vi "New from MsgPack bytes.vi"(8 "error in (no error)":errorcluster, 11 "Bytes in":u8[](array[numeric]) format="%x") -> (0 "error out":errorcluster, 2 "MsgPackExt":refnum<class "MsgPackExt.lvclass">, 3 "remaining bytes":u8[](array[numeric]))   [LabVIEW 2020, in "MessagePack.lvlib" / "MsgPackExt.lvclass"]
uses:
  MsgPackExt.lvclass
  MsgPackExt.lvclass/MsgPackExt.ctl
  <vilib>/Utility/error.llb/Error Cluster From Error Code.vi
  <vilib>/ErrorRing/Error Ring.xnode
  MessagePack.lvlib
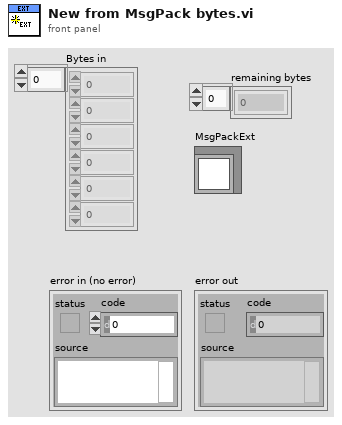
[diagram p1: front panel]
types:
  T1 = typedef "MessagePack.lvlib/MsgPack Object Types.ctl" = enum16{"UNSUPPORTED", "POSINT", "NEGINT", "FIXMAP", "FIXARRAY", "FIXSTR", "NIL", "FALSE", "TRUE", "BIN8", "BIN16", "BIN32", "EXT8", "EXT16", "EXT32", "FLOAT32", "FLOAT64", "UINT8", "UINT16", "UINT32", "UINT64", "INT8", "INT16", "INT32", "INT64", "FIXEXT1", "FIXEXT2", "FIXEXT4", "FIXEXT8", "FIXEXT16", "STR8", "STR16", "STR32", "ARRAY16", "ARRAY32", "MAP16", "MAP32"}
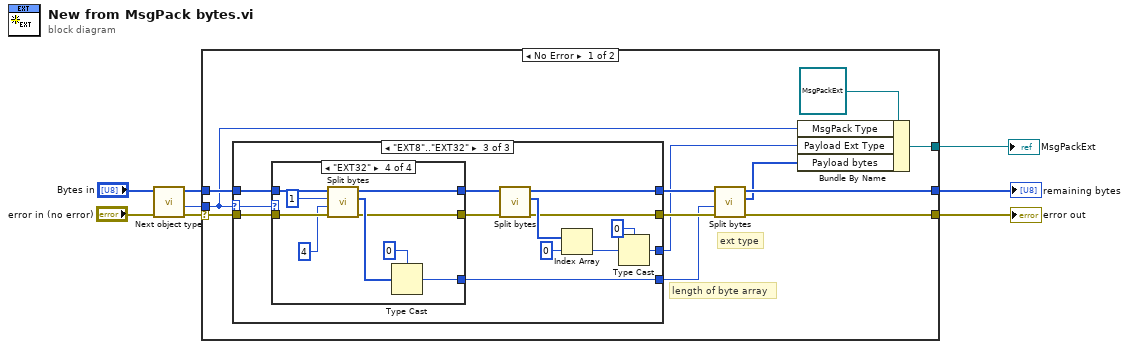
[diagram p0: block diagram]
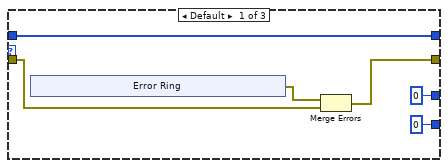
[diagram p2: hidden frame]
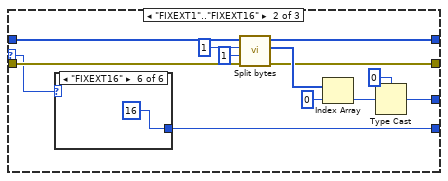
[diagram p3: hidden frame]
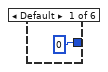
[diagram p4: hidden frame]
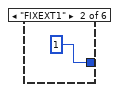
[diagram p5: hidden frame]
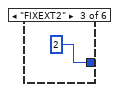
[diagram p6: hidden frame]
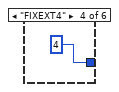
[diagram p7: hidden frame]
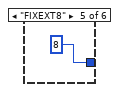
[diagram p8: hidden frame]
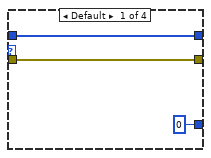
[diagram p9: hidden frame]
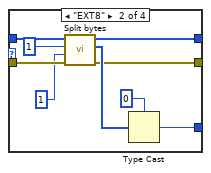
[diagram p10: hidden frame]
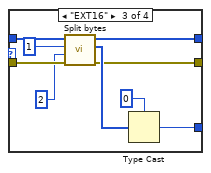
[diagram p11: hidden frame]
diagram:
  n1 = call "Next object type.vi"("error in (no error)"="error in (no error)", "Bytes in"="Bytes in") -> ("error out"=w6:errorcluster, "MsgPack Type"=w5:T1, "Bytes out"=w4:u8[])  [unwired: 6 in, 1 out]
  n2 = case shown="No Error" w6 {
    selector: w6 -> [w20 w94]
    tunnel: w5 -> [w9 _]
    tunnel: w4 -> [w19 w93]
    tunnel: [w15 w93] -> w3
    tunnel: [w14 w94] -> w1
    tunnel: [w12 _] -> w2
    frame No Error {
      # "length of byte array"
      # "ext type"
      n3 = case shown="\"EXT8\"..\"EXT32\"" w9 {
        selector: w9 -> [_ w33 w50]
        tunnel: w20 -> [w26 w41 w61]
        tunnel: [w24 w36 w56] -> w17
        tunnel: w19 -> [w23 w43 w62]
        tunnel: [w23 w35 w51] -> w18
        tunnel: [i8 0 w34 w53] -> w11
        tunnel: [u32 0 ("Count") w31 w52] -> w16
        frame Default {
          n4 = xnode "Error Ring"() -> ("error out"=w25:errorcluster)
          n5 = Merge Errors(w25, w26) -> (w24:errorcluster)
        }
        frame "FIXEXT1".."FIXEXT16" {
          n6 = case shown="\"FIXEXT16\"" w33 {
            tunnel: [u32 0 ("Count") u32 1 ("Count") u32 2 ("Count") u32 4 ("Count") u32 8 ("Count") u32 16 ("Count")] -> w31
            frame Default {
            }
            frame "FIXEXT1" {
            }
            frame "FIXEXT2" {
            }
            frame "FIXEXT4" {
            }
            frame "FIXEXT8" {
            }
            frame "FIXEXT16" {
            }
          }
          n7 = call "Split bytes.vi"("error in"=w41, "count (1)"=1 ("Count"), "start index (0)"=1 ("Start index"), "bytes in"=w43) -> ("error out"=w36:errorcluster, "selected bytes"=w39:u8[], "remaining bytes"=w35:u8[])  [unwired: 4 in, 1 out]
          n8 = Index Array(array=w39, index=0) -> (element=w37:u8)
          n9 = Type Cast(type=i8 0, x=w37) -> (*(type *) &x=w34:i8)
        }
        frame "EXT8".."EXT32" {
          n10 = case shown="\"EXT32\"" w50 {
            tunnel: w62 -> [w64 w74 w83 w92]
            tunnel: w61 -> [w65 w72 w81 w90]
            tunnel: [w65 w69 w78 w87] -> w60
            tunnel: [w64 w68 w77 w86] -> w59
            tunnel: [u32 0 w67 w76 w85] -> w52
            frame Default {
            }
            frame "EXT8" {
              n11 = call "Split bytes.vi"("error in"=w72, "count (1)"=1, "start index (0)"=1 ("Start index"), "bytes in"=w74) -> ("error out"=w69:errorcluster, "selected bytes"=w70:u8[], "remaining bytes"=w68:u8[])  [unwired: 4 in, 1 out]
              n12 = Type Cast(type=u8 0, x=w70) -> (*(type *) &x=w67:u8)
            }
            frame "EXT16" {
              n13 = call "Split bytes.vi"("error in"=w81, "count (1)"=2, "start index (0)"=1 ("Start index"), "bytes in"=w83) -> ("error out"=w78:errorcluster, "selected bytes"=w79:u8[], "remaining bytes"=w77:u8[])  [unwired: 4 in, 1 out]
              n14 = Type Cast(type=u16 0, x=w79) -> (*(type *) &x=w76:u16)
            }
            frame "EXT32" {
              n15 = call "Split bytes.vi"("error in"=w90, "count (1)"=4, "start index (0)"=1 ("Start index"), "bytes in"=w92) -> ("error out"=w87:errorcluster, "selected bytes"=w88:u8[], "remaining bytes"=w86:u8[])  [unwired: 4 in, 1 out]
              n16 = Type Cast(type=u32 0, x=w88) -> (*(type *) &x=w85:u32)
            }
          }
          n17 = call "Split bytes.vi"("error in"=w60, "bytes in"=w59) -> ("error out"=w56:errorcluster, "selected bytes"=w58:u8[], "remaining bytes"=w51:u8[])  [unwired: 6 in, 1 out]
          n18 = Index Array(array=w58, index=0) -> (element=w54:u8)
          n19 = Type Cast(type=i8 0, x=w54) -> (*(type *) &x=w53:i8)
        }
      }
      n20 = call "Split bytes.vi"("error in"=w17, "count (1)"=w16, "bytes in"=w18) -> ("error out"=w14:errorcluster, "selected bytes"=w10:u8[], "remaining bytes"=w15:u8[])  [unwired: 5 in, 1 out]
      n21 = Bundle By Name(cluster=refnum<class "MsgPackExt.lvclass"> refnum ("MessagePack.lvlib:MsgPackExt.lvclass"), "MsgPack Type"=w9, "Payload Ext Type"=w11, "Payload bytes"=w10) -> (w12:refnum<class "MsgPackExt.lvclass">)
    }
    frame Error {
    }
  }
  "error out" <- w1
  "MsgPackExt" <- w2
  "remaining bytes" <- w3
